vi "Regex Test.vi"() -> ()   [LabVIEW 2018]
uses:
  Failure Information.ctl
  Log Record.ctl
  Logger/Internal Log Levels.ctl
  Filters/Aggregation Method.ctl
  Filters/Match Behavior.ctl
  40037e18-95a9-4cb9-9ddf-d3c11cbaea1d.vi
  40037e18-95a9-4cb9-9ddf-d3c11cbaea1d.vi/a153a250-4fb8-4a99-bb5b-6ccb57f1f631.vi
  40037e18-95a9-4cb9-9ddf-d3c11cbaea1d.vi/a153a250-4fb8-4a99-bb5b-6ccb57f1f631.vi/28727e37-b0d9-407c-a479-ab0b7779cd69.vi
  Filters/Regex/Regex.lvclass
  C:/Users/Colin/Documents/software_projects/glog/Logging/Filters/Filter/Filter.lvclass
  Handlers/File Handler/File Handler.lvclass
  C:/Users/Colin/Documents/software_projects/glog/Logging/Handlers/Formatting Handler/Formatting Handler.lvclass
  Filters/Regex/New (Element).vi
  Filters/Regex/New (Array).vi
  Registry/Log.vi
  Logging.lvlib
panel:
  out "failures info":T1[](array[typedef]) {"Log Record"."timestamp" format="%<%x %.3X>T"}
  out "error out":errorcluster
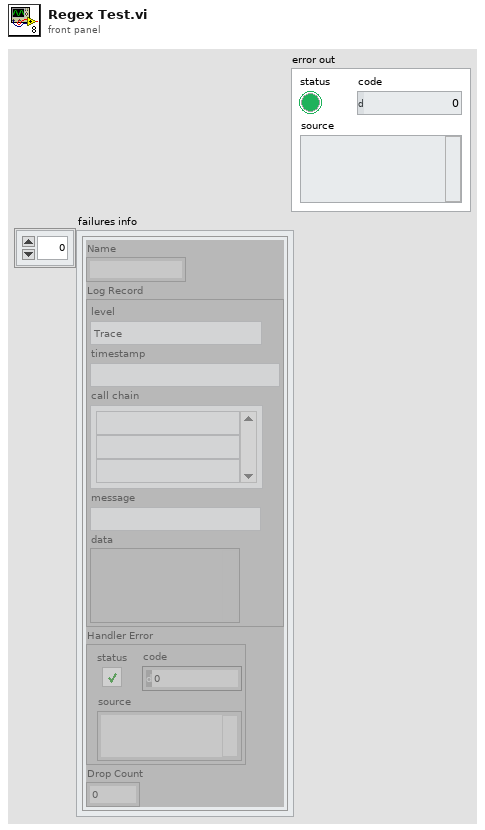
[diagram p1: front panel]
types:
  T1 = typedef "Logging.lvlib/Failure Information.ctl" = cluster{"Name":string, "Log Record":T2, "Handler Error":errorcluster, "Drop Count":u32}
  T2 = typedef "Logging.lvlib/Log Record.ctl" = cluster{"level":T3, "timestamp":timestamp, "call chain":string[], "message":string, "data":variant}
  T3 = typedef "Logging.lvlib/Internal Log Levels.ctl" = enum16{"Trace", "Debug", "Info", "Warning", "Error", "Critical", "Internal"}
  T4 = typedef "Logging.lvlib/Match Behavior.ctl" = enum16{"Keep", "Discard"}
  T5 = typedef "Logging.lvlib/Aggregation Method.ctl" = enum16{"Any", "Only", "All", "None"}
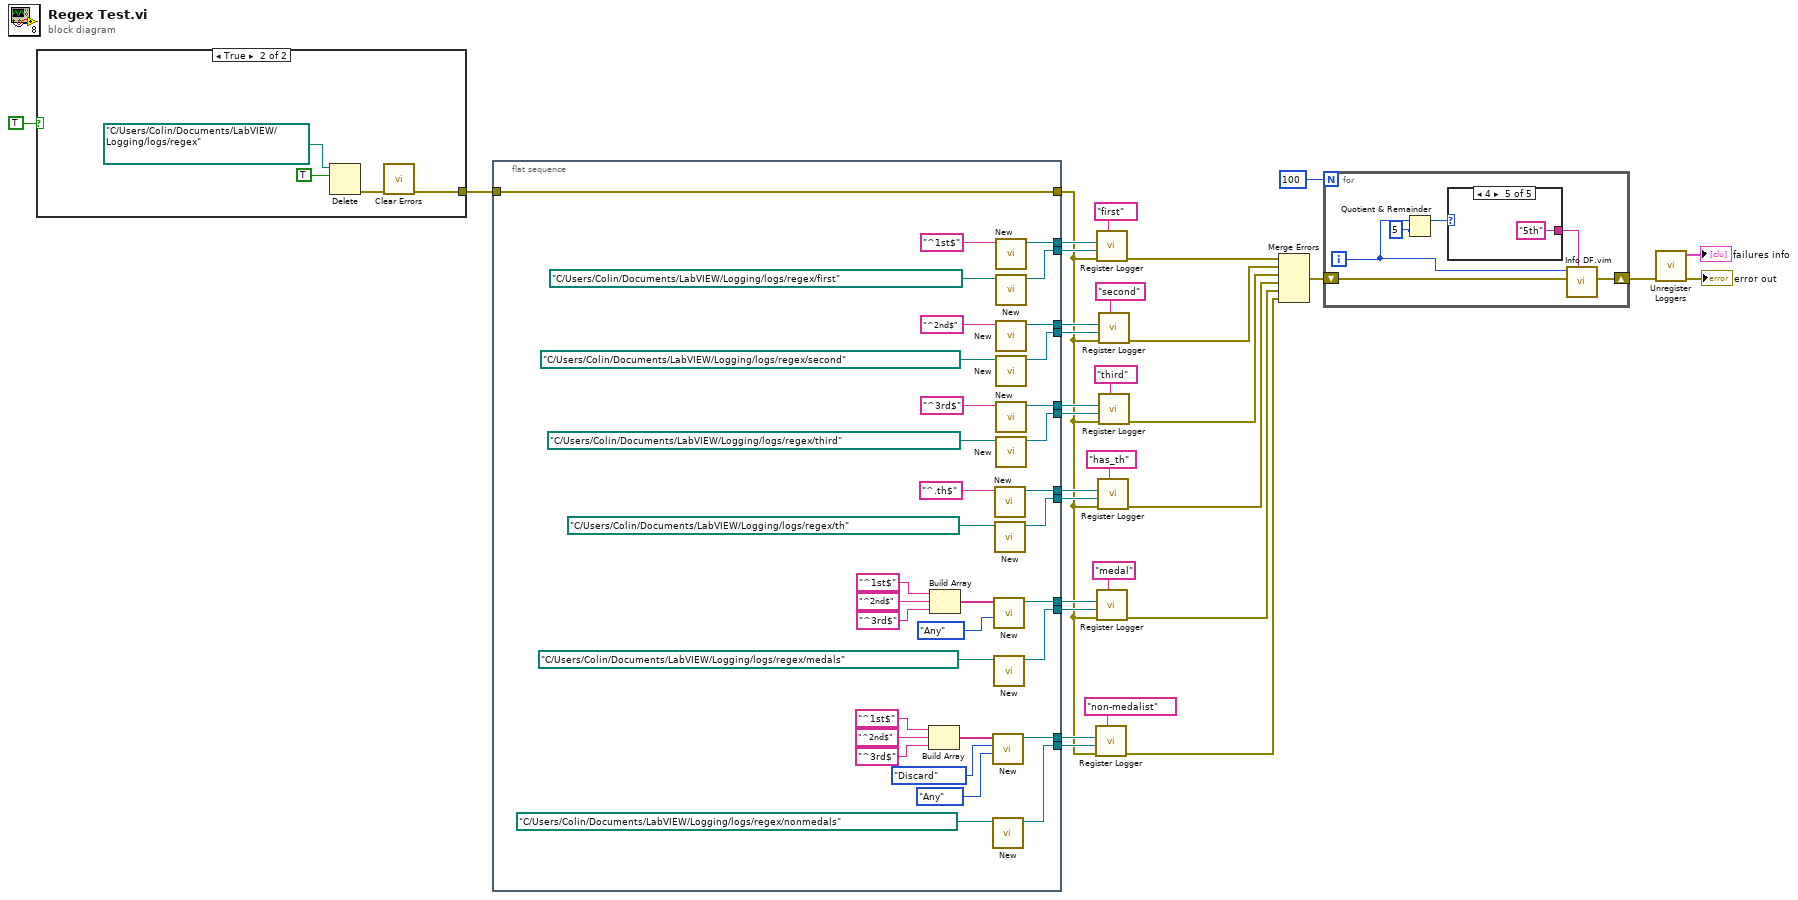
[diagram p0: block diagram]
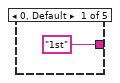
[diagram p3: hidden frame]
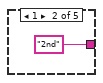
[diagram p4: hidden frame]
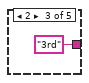
[diagram p5: hidden frame]
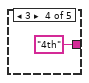
[diagram p6: hidden frame]
diagram:
  n1 = case shown="True" TRUE {
    tunnel: [_ w36] -> w21
    frame False {
    }
    frame True {
      n2 = Delete(path (use dialog)=path "C:/Users/Colin/Documents/LabVIEW/Logging/logs/regex" ("log directory (<app dir>/logs)"), entire hierarchy (F)=TRUE) -> (error out=w34:errorcluster)  [unwired: 3 in, 2 out]
      n3 = call <vilib>:"Clear Errors.vi"("error in (no error)"=w34) -> ("error out"=w36:errorcluster)  [unwired: 5 in, 1 out]
    }
  }
  n4 = flat-sequence {
    tunnel: [w70] -> w32
    tunnel: [w68] -> w31
    tunnel: [w67] -> w30
    tunnel: [w65] -> w29
    tunnel: w21 -> [w62]
    tunnel: [w62] -> w4
    tunnel: [w58] -> w18
    tunnel: [w60] -> w19
    tunnel: [w57] -> w16
    tunnel: [w55] -> w15
    tunnel: [w51] -> w10
    tunnel: [w52] -> w11
    tunnel: [w40] -> w7
    tunnel: [w39] -> w6
    frame #0 {
      n5 = Build Array("^1st$" ("regex string"), "^2nd$" ("regex string"), "^3rd$" ("regex string")) -> (w44:string[])
      n6 = Build Array("^1st$" ("regex string"), "^2nd$" ("regex string"), "^3rd$" ("regex string")) -> (w47:string[])
      n7 = call-poly "New.vi"("aggregation method (all)"=Aggregation_Method."Any", "match behavior (keep)"=Match_Behavior."Discard", "regex strings"=w44) -> ("regex out"=w39:refnum<class "Regex.lvclass">)  [unwired: 7 in, 1 out]
      n8 = call "New.vi"("log directory (<app dir>/logs)"=path "C:/Users/Colin/Documents/LabVIEW/Logging/logs/regex/nonmedals") -> ("file handler"=w40:refnum<class "File Handler.lvclass">)  [unwired: 10 in]
      n9 = call-poly "New.vi"("aggregation method (all)"=Aggregation_Method."Any", "regex strings"=w47) -> ("regex out"=w52:refnum<class "Regex.lvclass">)  [unwired: 8 in, 1 out]
      n10 = call "New.vi"("log directory (<app dir>/logs)"=path "C:/Users/Colin/Documents/LabVIEW/Logging/logs/regex/medals") -> ("file handler"=w51:refnum<class "File Handler.lvclass">)  [unwired: 10 in]
      n11 = call-poly "New.vi"("regex string"="^.th$") -> ("regex out"=w55:refnum<class "Regex.lvclass">)  [unwired: 9 in, 1 out]
      n12 = call "New.vi"("log directory (<app dir>/logs)"=path "C:/Users/Colin/Documents/LabVIEW/Logging/logs/regex/th") -> ("file handler"=w57:refnum<class "File Handler.lvclass">)  [unwired: 10 in]
      n13 = call-poly "New.vi"("regex string"="^1st$") -> ("regex out"=w70:refnum<class "Regex.lvclass">)  [unwired: 9 in, 1 out]
      n14 = call "New.vi"("log directory (<app dir>/logs)"=path "C:/Users/Colin/Documents/LabVIEW/Logging/logs/regex/first") -> ("file handler"=w68:refnum<class "File Handler.lvclass">)  [unwired: 10 in]
      n15 = call-poly "New.vi"("regex string"="^2nd$") -> ("regex out"=w65:refnum<class "Regex.lvclass">)  [unwired: 9 in, 1 out]
      n16 = call "New.vi"("log directory (<app dir>/logs)"=path "C:/Users/Colin/Documents/LabVIEW/Logging/logs/regex/second") -> ("file handler"=w67:refnum<class "File Handler.lvclass">)  [unwired: 10 in]
      n17 = call-poly "New.vi"("regex string"="^3rd$") -> ("regex out"=w60:refnum<class "Regex.lvclass">)  [unwired: 9 in, 1 out]
      n18 = call "New.vi"("log directory (<app dir>/logs)"=path "C:/Users/Colin/Documents/LabVIEW/Logging/logs/regex/third") -> ("file handler"=w58:refnum<class "File Handler.lvclass">)  [unwired: 10 in]
    }
  }
  n19 = call "Register Logger.vi"("name (\"Default\")"="non-medalist" ("name (\"Default\")"), "error in (no error)"=w4, "log handler (file handler)"=w7, "log filter (none)"=w6) -> ("error out"=w5:errorcluster)  [unwired: 7 in]
  n20 = call "Register Logger.vi"("name (\"Default\")"="first" ("name (\"Default\")"), "error in (no error)"=w4, "log handler (file handler)"=w31, "log filter (none)"=w32) -> ("error out"=w27:errorcluster)  [unwired: 7 in]
  n21 = call "Register Logger.vi"("name (\"Default\")"="medal" ("name (\"Default\")"), "error in (no error)"=w4, "log handler (file handler)"=w10, "log filter (none)"=w11) -> ("error out"=w12:errorcluster)  [unwired: 7 in]
  n22 = call "Register Logger.vi"("name (\"Default\")"="has_th" ("name (\"Default\")"), "error in (no error)"=w4, "log handler (file handler)"=w16, "log filter (none)"=w15) -> ("error out"=w14:errorcluster)  [unwired: 7 in]
  n23 = call "Register Logger.vi"("name (\"Default\")"="second" ("name (\"Default\")"), "error in (no error)"=w4, "log handler (file handler)"=w30, "log filter (none)"=w29) -> ("error out"=w28:errorcluster)  [unwired: 7 in]
  n24 = call "Register Logger.vi"("name (\"Default\")"="third" ("name (\"Default\")"), "error in (no error)"=w4, "log handler (file handler)"=w18, "log filter (none)"=w19) -> ("error out"=w20:errorcluster)  [unwired: 7 in]
  n25 = Merge Errors(w27, w28, w20, w14, w12, w5) -> (w24:errorcluster)
  n26 = for {
    N: 100 -> [_]
    shift-right: [w74] -> w3
    shift-left: w24 -> [w75]
    i -> [w73]
    n27 = Quotient & Remainder(x=w73, y=5) -> (x-y*floor(x/y)=w71:i32)  [unwired: 1 out]
    n28 = case shown="4" w71 {
      tunnel: ["1st" ("message") "2nd" ("message") "3rd" ("message") "4th" ("message") "5th" ("message")] -> w76
      frame 0, Default {
      }
      frame 1 {
      }
      frame 2 {
      }
      frame 3 {
      }
      frame 4 {
      }
    }
    n29 = call "Info DF.vim"("message"=w76, "dataflow in"=w75, "data (null)"=w73) -> ("dataflow out"=w74:errorcluster)  [unwired: 8 in]
  }
  n30 = call "Unregister Loggers.vi"("error in (no error)"=w3) -> ("error out"=→"error out":errorcluster, "failures info"=→"failures info":T1[])  [unwired: 9 in]
